vi "Initialize.vi"(8 "error in (no error)":errorcluster) -> (0 "error out":errorcluster, 1 "Exit Event out":refnum<user-event>, 2 "queue out":refnum<queue>, 3 "Event Registration Refnum out":refnum<event-registration>)   [LabVIEW 2026, in "VILab.lvlib" / "FaKI State Machine.lvlib"]
doc: "Initializes and registers for the \"Exit\" user event. Initializes the queue and enqueues the \"Macro: Initialize\" state.\n\nThis VI is inlined."
uses:
  FaKI State Machine.lvlib
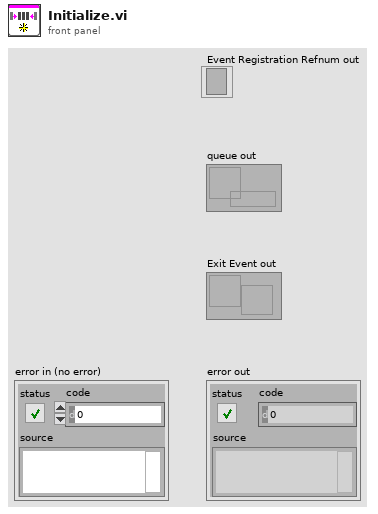
[diagram p1: front panel]
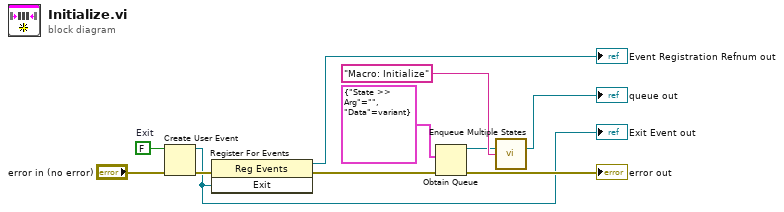
[diagram p0: block diagram]
diagram:
  w7 = FALSE  # Exit
  n1 = Create User Event(user event datatype=w7, error in="error in (no error)") -> (user event=w1:refnum<user-event>, error out=w8:errorcluster)
  "Exit Event out" <- w1
  n2 = register-events(error in=w8, w1) -> (reference out=→"Event Registration Refnum out":refnum<event-registration>, error out=w6:errorcluster)  [unwired: 1 in]
  n3 = Obtain Queue(element data type=cluster{"State >> Arg":string, "Data":variant} {"State >> Arg"="", "Data"=variant}, error in (no error)=w6) -> (queue out=w9:refnum<queue>, error out=→"error out":errorcluster)  [unwired: 3 in, 1 out]
  n4 = call "Enqueue Multiple States.vi"("queue in"=w9, "State(s) at Back"="Macro: Initialize") -> ("queue out"=→"queue out":refnum<queue>)  [unwired: 13 in]
